vi "Acquire AVI.vi"() -> ()   [LabVIEW 2021]
panel:
  in  "Gest":string="fist"
  in  "Test":bool
  out "Frame Rate":dbl
  out "error out":errorcluster
  in  "Stop (F)":bool
  out "Image Out":T1(plugin-control)
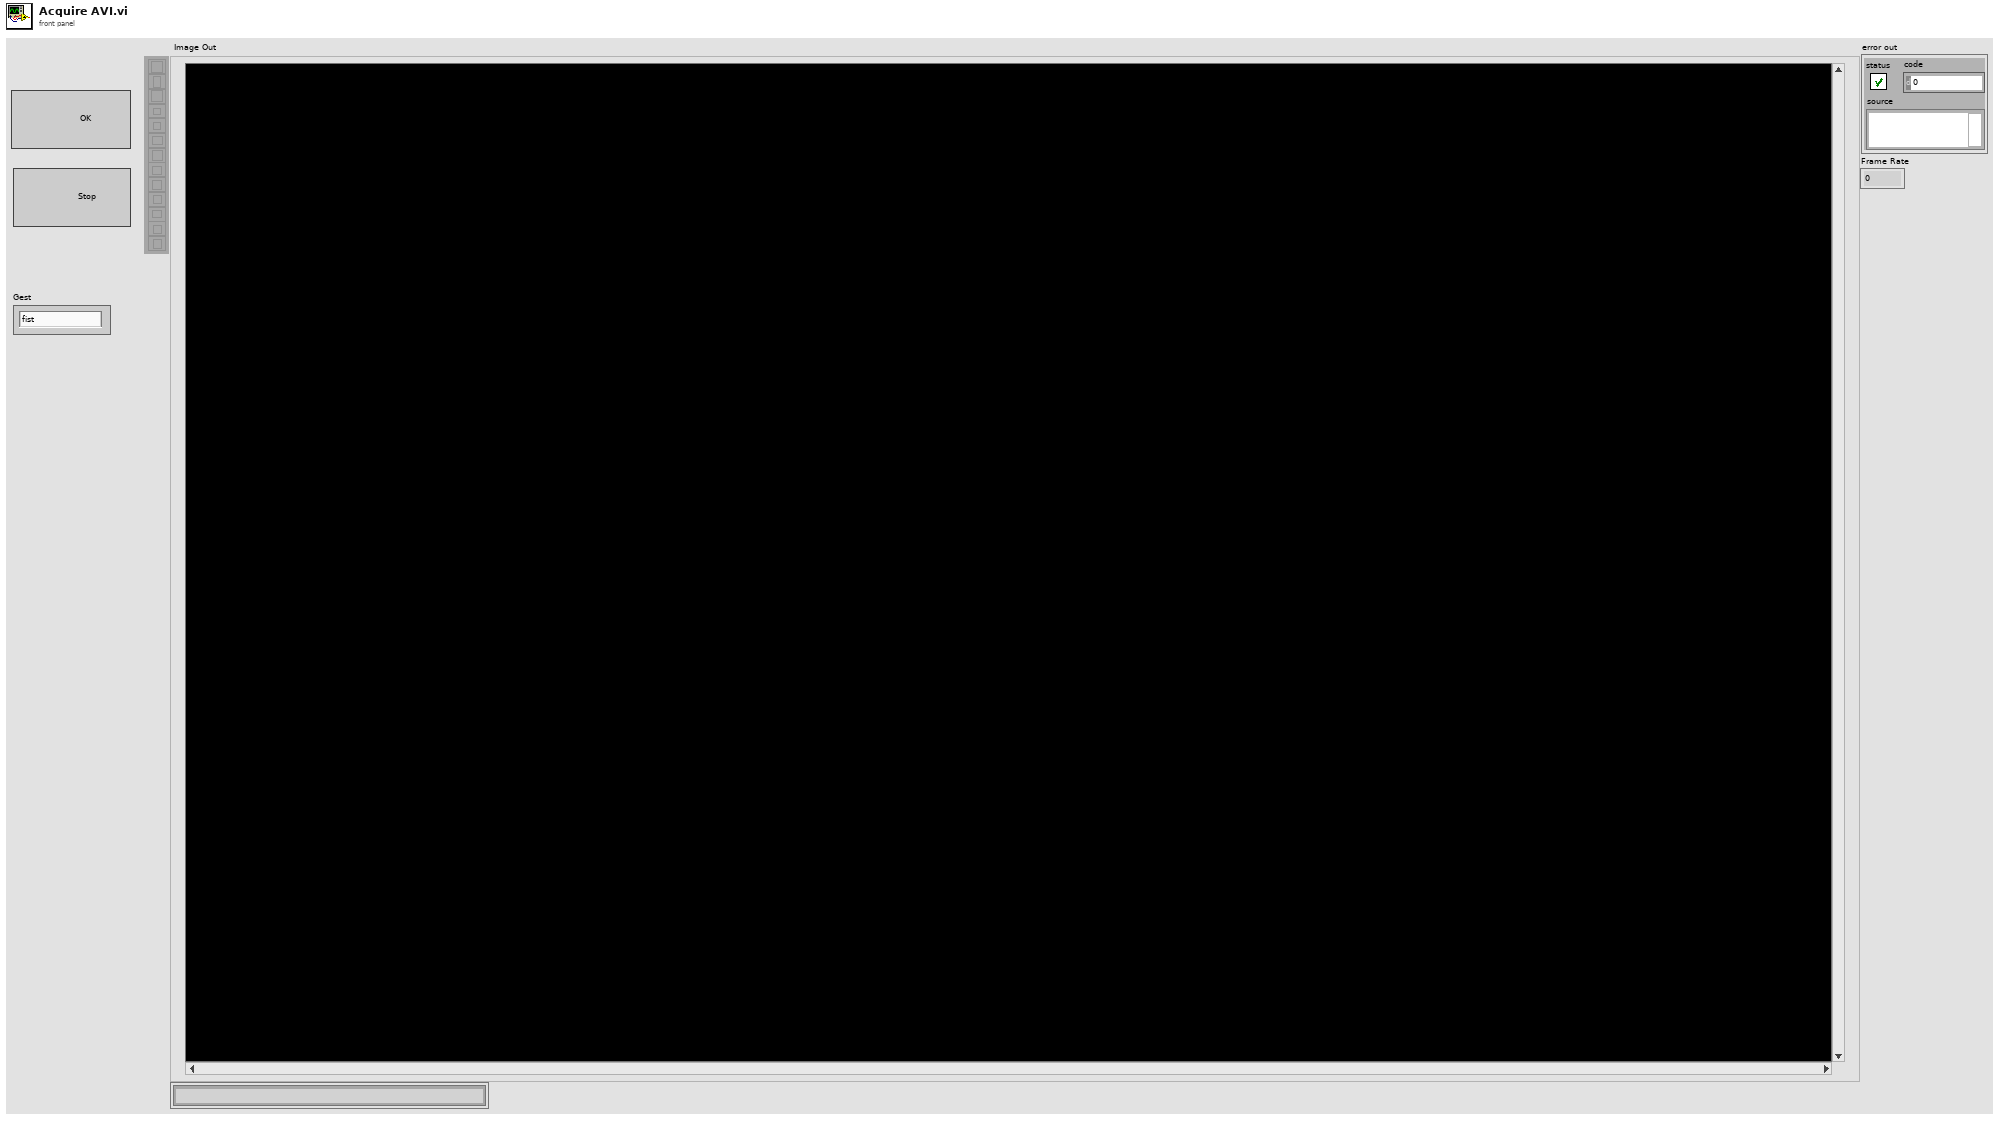
[diagram p1: front panel]
types:
  T1 = typedef "IMAQ Image.ctl" = refnum<image>
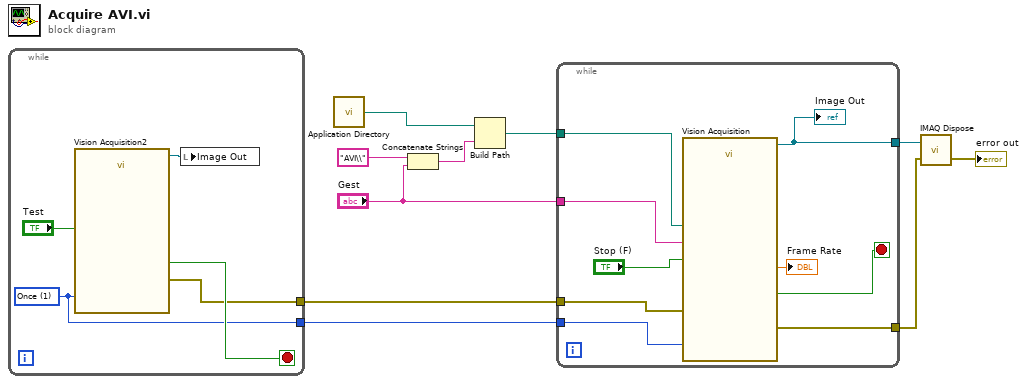
[diagram p0: block diagram]
diagram:
  n1 = while {
    tunnel: [w12] -> w8
    tunnel: [w11] -> w4
    stop <- w13 stop-if-true
    w11 = u32 1 items=["Off", "Once"] ("Balance White Auto")
    n2 = call "Vision Acquisition2"("Balance White Auto"=w11, "Stop (F)"="Test") -> ("Image Out"=w15:T1, "Stopped"=w13:bool, "error out"=w12:errorcluster)  [unwired: 22 in, 1 out]
    n3 = local write "Image Out"(w15) -> ()
  }
  n4 = call <vilib>:"Application Directory.vi"() -> ("Application Directory"=w10:path)
  n5 = Concatenate Strings("AVI\\", "Gest") -> (w6:string)
  n6 = Build Path(base path=w10, name or relative path=w6) -> (appended path=w9:path)
  n7 = while {
    tunnel: w9 -> [w21]
    tunnel: w8 -> [w20]
    tunnel: "Gest" -> [w19]
    tunnel: w4 -> [w18]
    tunnel: [w17] -> w3
    tunnel: [w16] -> w2
    stop <- w23 stop-if-true
    n8 = call "Vision Acquisition"("Image Logging Path"=w21, "Image Logging Prefix"=w19, "Balance White Auto"=w18, "Stop (F)"="Stop (F)", "error in"=w20) -> ("Image Out"=w17:T1, "Frame Rate"=→"Frame Rate":dbl, "Stopped"=w23:bool, "error out"=w16:errorcluster)  [unwired: 19 in]
    "Image Out" <- w17
  }
  n9 = call "IMAQ Dispose"("Image"=w3, "error in (no error)"=w2) -> ("error out"=→"error out":errorcluster)  [unwired: 4 in]
